vi "UsrProfiles-Save with options.vi"(8 "error in":errorcluster) -> (0 "error out":errorcluster)   [LabVIEW 2020]
uses:
  Typedefs/Which path.ctl
  Globals/gl_UsrProfiles globals.vi
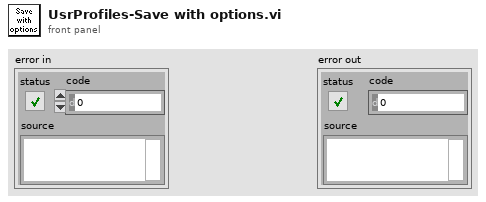
[diagram p1: front panel]
types:
  T1 = typedef "Which path.ctl" = enum16{"Configuration Files", "Calibration Files", "Images", "Setup.ini", "Loaded User profile.ini", "User's-Previous session.ini", "New user profile.ini", "Selected User profile.ini", "User profiles folder", "Power meter scaling.txt", "FOV Cal.ini", "Calibration.ini"}
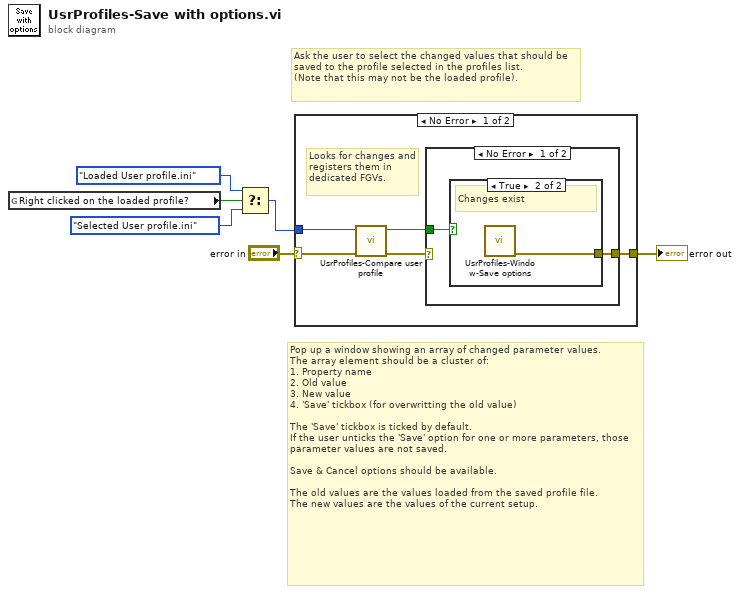
[diagram p0: block diagram]
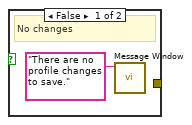
[diagram p2: hidden frame]
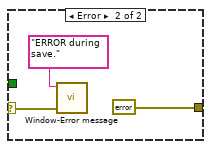
[diagram p3: hidden frame]
diagram:
  # "Ask the user to select the changed values that should be saved to the profile selected in the profiles list.\n(Note that this may not be the loaded profile)."
  # "Pop up a window showing an array of changed parameter values.\nThe array element should be a cluster of:\n1. Property name\n2. Old value\n3. New value\n4. 'Save' tickbox (for overwritting the old value)\n\nThe 'Save' tickbox is ticked by default.\nIf the user unticks the 'Save' option for one or more parameters, those parameter values are not saved.\n\nSave & Cancel options should be available.\n\nThe old values are the values loaded from the saved profile file.\nThe new values are the values of the current setup."
  n1 = global read "gl_UsrProfiles globals.vi" "Right clicked on the loaded profile?"() -> (w3:bool)
  n2 = Select(t=Which_path."Loaded User profile.ini" ("Which file?"), s=w3, f=Which_path."Selected User profile.ini" ("Which file?")) -> (s? t:f=w1:T1)
  n3 = case shown="No Error" "error in" {
    selector: "error in" -> [w11 w19]
    tunnel: [w10 w19] -> w5
    tunnel: w1 -> [w7 _]
    frame No Error {
      # "Looks for changes and registers them in dedicated FGVs."
      n4 = call "UsrProfiles-Compare user profile.vi"("error in"=w11, "Which profile?"=w7) -> ("error out"=w8:errorcluster, "Changes exist"=w9:bool)  [unwired: 8 in]
      n5 = case shown="No Error" w8 {
        selector: w8 -> [_ w18]
        tunnel: [w13 errorcluster {"status"=FALSE, "code"=0, "source"=""} ("error out")] -> w10
        tunnel: w9 -> [w12 _]
        frame No Error {
          n6 = case shown="True" w12 {
            tunnel: [_ w15] -> w13
            frame False {
              # "No changes"
              n7 = call "Message Window.vi"("Message string"="There are no profile changes to save.") -> ()  [unwired: 10 in, 1 out]
            }
            frame True {
              # "Changes exist"
              n8 = call "UsrProfiles-Window-Save options.vi"() -> ("error out"=w15:errorcluster)  [unwired: 10 in, 1 out]
            }
          }
        }
        frame Error {
          n9 = call "Window-Error message.vi"("error in (no error)"=w18, "Message"="ERROR during save.") -> ()  [unwired: 9 in, 1 out]
        }
      }
    }
    frame Error {
    }
  }
  "error out" <- w5
